vi "Stop Core.vi"(10 "final error code":i32, 11 "AMS Gas Actor in":refnum<class "AMS Gas Actor.lvclass">) -> (3 "AMS Gas Actor out":refnum<class "AMS Gas Actor.lvclass">)   [LabVIEW 2015, in "AMS UI.lvlib" / "AMS Gas Actor.lvclass"]
doc: "(<B>Filename</B>: Actor Framework.lvlib:Actor.lvclass:Stop Core.vi)\n\nDefines what the actor does before it stops. Use the <B>final error code</B> input to determine whether the actor shut down in response to an error.\n\nBy default, this method does nothing. A descendant class may override it to define behavior, such as shutting down any processes the actor initiated in its override of the Actor Core method."
uses:
  AMS Gas Actor.lvclass
  AMS Gas Actor.lvclass/AMS Gas Actor.ctl
  eActor/eActor.lvclass
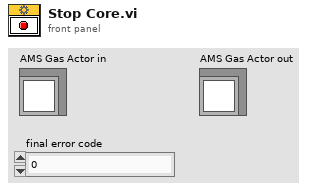
[diagram p1: front panel]
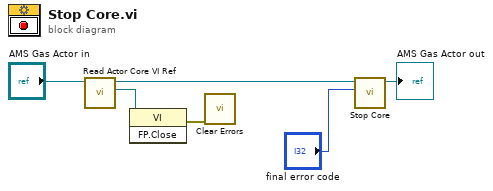
[diagram p0: block diagram]
diagram:
  n1 = call "Read Actor Core VI Ref.vi"("AMS Gas Actor in"="AMS Gas Actor in") -> ("Actor Core VI Ref"=w1:refnum<vi>, "AMS Gas Actor out"=w3:refnum<class "AMS Gas Actor.lvclass">)  [unwired: 9 in]
  n2 = invoke class="VI" method="FP.Close"(reference=w1) -> (error out=w2:errorcluster)  [unwired: 2 in, 2 out]
  n3 = call <vilib>:"Clear Errors.vi"("error in (no error)"=w2) -> ()  [unwired: 5 in, 2 out]
  n4 = call-parent "Stop Core.vi"("final error code"="final error code", "eActor in"=w3) -> ("eActor out"=→"AMS Gas Actor out":refnum<class "AMS Gas Actor.lvclass">)  [unwired: 9 in]
